vi "Chain Reaction.vi"(0 "1D Board":T1[](array[typedef]), 5 "Team Number":i32, 11 "error in (no error)":errorcluster) -> (4 "1D Board Out":T1[](array[typedef]), 6 "Won?":bool, 8 "Coins Won":i32, 15 "error out":errorcluster)   [LabVIEW 2014, in "Dragon Tamers.lvlib"]
uses:
  Dragon Tamers.lvlib
  Typedefs/Board Cell.ctl
  Typedefs/Cell Occupancy.ctl
  <userlib>/_OpenG.lib/array/array.llb/Filter 1D Array with Scalar (Boolean)__ogtk.vi
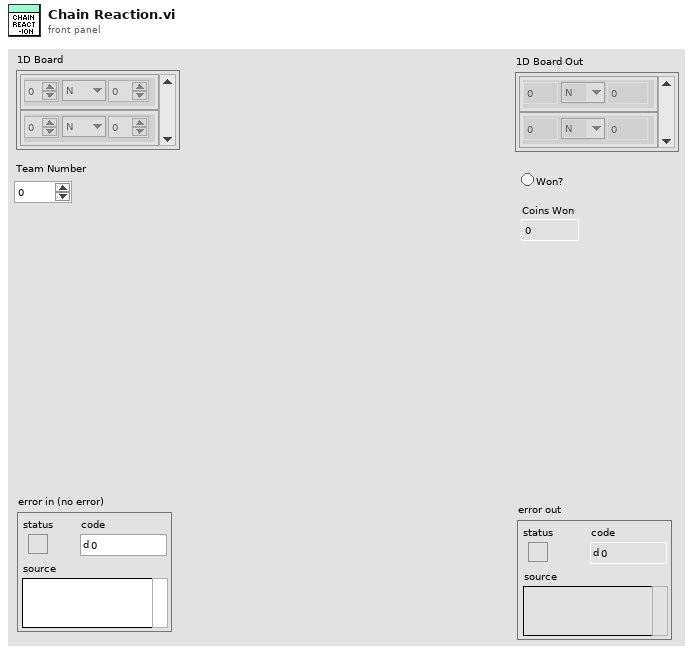
[diagram p1: front panel]
types:
  T1 = typedef "Dragon Tamers.lvlib/Board Cell.ctl" = cluster{"Team":i32, "Occu.":T2, "Count":i32}
  T2 = typedef "Dragon Tamers.lvlib/Cell Occupancy.ctl" = enum16{"N", "C", "K"}
  T3 = typedef "Dragon Tamers.lvlib/Parsed Board.ctl" = cluster{"DT King":i32, "Opp King":i32, "Count":i32[], "Empty Cells":i32[], "DT Cells":i32[], "Opp Cells":i32[], "DT Team":i32, "Opp. Team":i32}
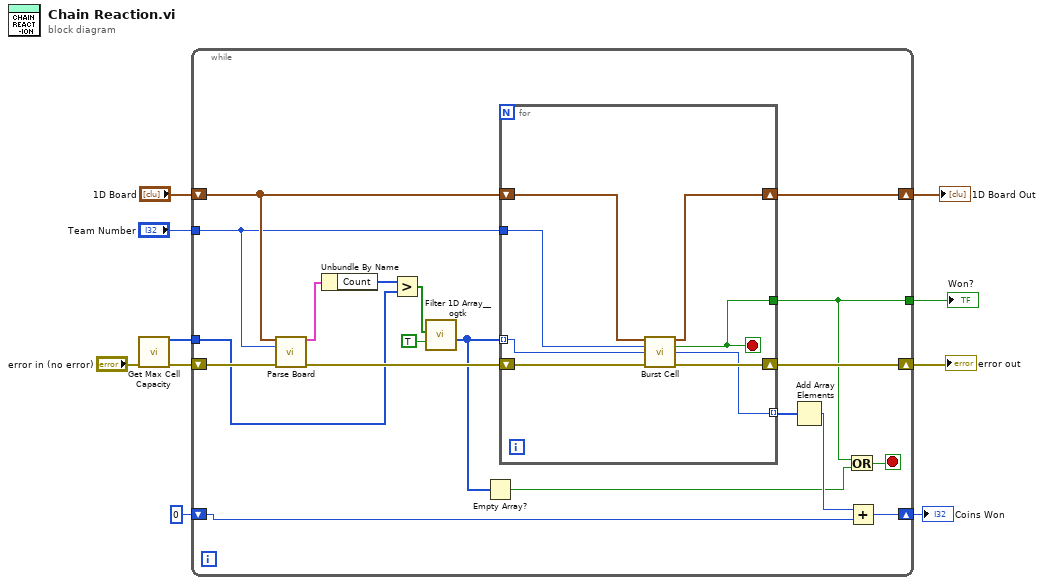
[diagram p0: block diagram]
diagram:
  n1 = call "Get Max Cell Capacity.vi"("error in (no error)"="error in (no error)") -> ("Max Capacity[]"=w4:i32[], "error out"=w5:errorcluster)  [unwired: 13 in]
  n2 = while {
    tunnel: "Team Number" -> [w19]
    shift-right: [w22] -> w8
    shift-left: "1D Board" -> [w23]
    shift-right: [w18] -> w7
    shift-left: w5 -> [w29]
    tunnel: w4 -> [w20]
    tunnel: [w13] -> w3
    shift-right: [w15] -> w1
    shift-left: 0 -> [w14]
    stop <- w11 stop-if-true
    n3 = call "Parse Board.vi"("Board Array"=w23, "DT Team #"=w19, "error in (no error)"=w29) -> ("Parsed Board Info"=w28:T3, "error out"=w26:errorcluster)  [unwired: 11 in]
    n4 = Unbundle By Name(w28) -> ("Count"=w27:i32[])
    n5 = Greater?(x=w27, y=w20) -> (0:w25:bool[])
    n6 = call-poly <userlib>:"Filter 1D Array__ogtk.vi"("items to filter"=TRUE, "array"=w25) -> ("filtered item indices"=w21:i32[])  [unwired: 4 in, 1 out]
    n7 = Empty Array?(array=w21) -> (empty?=w12:bool)
    n8 = for {
      tunnel: w21 -> [w37] mode=indexing
      shift-right: [w34] -> w22
      shift-left: w23 -> [w35]
      shift-right: [w32] -> w18
      shift-left: w26 -> [w33]
      tunnel: w19 -> [w36]
      tunnel: [w31] -> w13
      tunnel: [w30] -> w17 mode=indexing
      stop <- w31 stop-if-true
      n9 = call "Burst Cell.vi"("1D Board"=w35, "Team Number"=w36, "Index to Burst"=w37, "error in (no error)"=w33) -> ("1D Board Out"=w34:T1[], "Won?"=w31:bool, "Coins Won"=w30:i32, "error out"=w32:errorcluster)  [unwired: 8 in]
    }
    n10 = Add Array Elements(numeric array=w17) -> (sum=w16:i32)
    n11 = Or(x=w13, y=w12) -> (x .or. y?=w11:bool)
    n12 = Add(x=w16, y=w14) -> (x+y=w15:i32)
  }
  "1D Board Out" <- w8
  "error out" <- w7
  "Won?" <- w3
  "Coins Won" <- w1
